vi "Digital Output User Interface.vi"() -> ()   [LabVIEW 2023, in "GUI.lvlib" / "Diagnostic.lvlib"]
uses:
  Diagnostic.lvlib
  Control/Digital Output 6514.ctl
  Control/Digital Output.ctl
  HardwareAbstractionLayer_LVOOP/Digital Output/NI Digital Output_class/NI Digital Output.lvclass
  D:/eDCU LTT/VT LTT Project/Source Code/HardwareAbstractionLayer_LVOOP/Digital Output/DO_class/DO.lvclass
  HardwareAbstractionLayer_LVOOP/Database/SQL Public VI/Control/DB Options.ctl
  HardwareAbstractionLayer_LVOOP/Main/Class Ref.ctl
  HardwareAbstractionLayer_LVOOP/DMM/DMM.lvclass
  HardwareAbstractionLayer_LVOOP/Function Generator/Function Generator.lvclass
  HardwareAbstractionLayer_LVOOP/Oscilloscope/Oscilloscope.lvclass
  HardwareAbstractionLayer_LVOOP/PowerSupply/PowerSupply.lvclass
  HardwareAbstractionLayer_LVOOP/Teststand/Teststand.lvclass
  HardwareAbstractionLayer_LVOOP/Analog Output/AO/AO.lvclass
  HardwareAbstractionLayer_LVOOP/Analog Input/AI/AI.lvclass
  HardwareAbstractionLayer_LVOOP/Database/Database.lvclass
  HardwareAbstractionLayer_LVOOP/Digital Output/DO_class/DO.lvclass
  HardwareAbstractionLayer_LVOOP/Digital Input/DI_class/DI.lvclass
  HardwareAbstractionLayer_LVOOP/PWM Output/PWM Output_class/PWM Output.lvclass
  HardwareAbstractionLayer_LVOOP/PWM Input/PWM Input_class/PWM Input.lvclass
  HardwareAbstractionLayer_LVOOP/NI Switch/NISwitch_class/NISwitch.lvclass
  HardwareAbstractionLayer_LVOOP/Modbus/Modbus_class/Modbus.lvclass
  HardwareAbstractionLayer_LVOOP/CAN/CAN Lib/CAN_class/CAN.lvclass
  HardwareAbstractionLayer_LVOOP/Main/Main.lvclass
  <userlib>/_OpenG.lib/appcontrol/appcontrol.llb/openg_application_control.lvlib
panel:
  in  "Start Acquire":bool
  in  "Stop Acquire":bool
  out "error out":errorcluster
  in  "error in":errorcluster
  in  "Operation":enum32{"6514-PXI2Slot9"}(tab)
  in  "PXIe_6514":T1
  in  "Stop":bool caption="Blank"
  in  "Apply":bool caption="Blank"
  # "Digital Output"
  # "Device:"
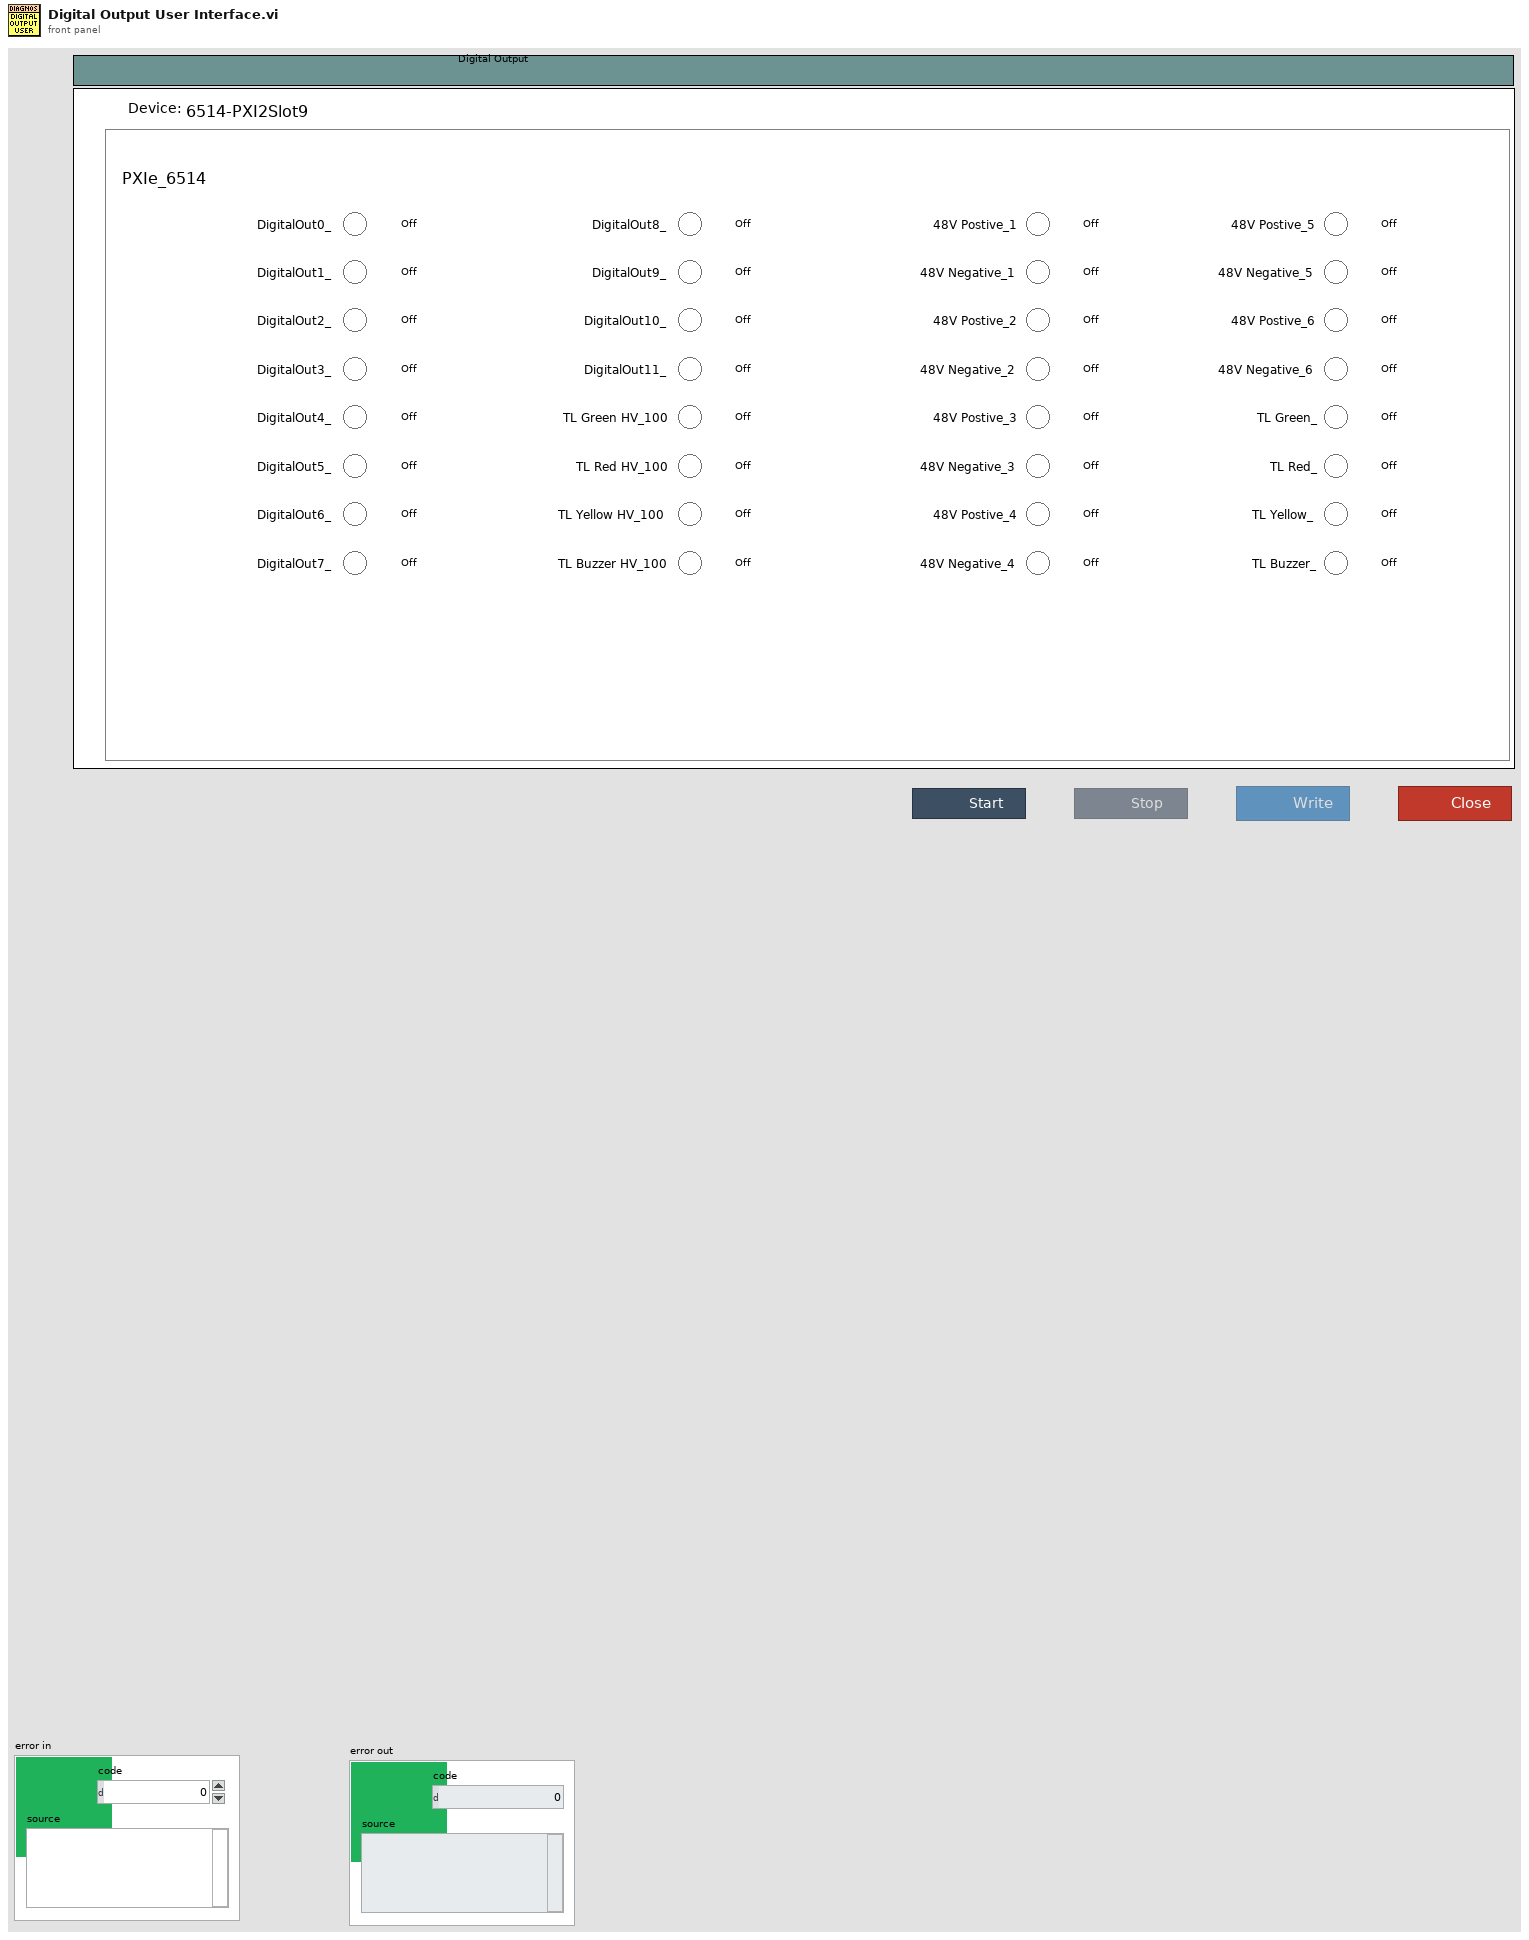
[diagram p1: front panel]
types:
  T1 = typedef "GUI.lvlib/Diagnostic.lvlib/Digital Output 6514.ctl" = cluster{"Channel-0":T2, "Channel-1":T2, "Channel-2":T2, "Channel-3":T2, "Channel-4":T2, "Channel-5":T2, "Channel-6":T2, "Channel-7":T2, "Channel-8":T2, "Channel-9":T2, "Channel-10":T2, "Channel-11":T2, "Channel-12":T2, "Channel-13":T2, "Channel-14":T2, "Channel-15":T2, "Channel-16":T2, "Channel-17":T2, "Channel-18":T2, "Channel-19":T2, "Channel-20":T2, "Channel-21":T2, "Channel-22":T2, "Channel-23":T2, "Channel-24":T2, "Channel-25":T2, "Channel-26":T2, "Channel-27":T2, "Channel-28":T2, "Channel-29":T2, "Channel-30":T2, "Channel-31":T2}
  T2 = typedef "GUI.lvlib/Diagnostic.lvlib/Digital Output.ctl" = bool
  T3 = typedef "HardwareAbstractionLayer_LVOOP.lvlib/Database.lvclass/DB Options.ctl" = enum16{"Init", "Select Data", "Insert Data", "Update Data", "Delete Data", "Execute Query", "Create Schema", "Create Table", "List Tables", "List Columns", "Close"}
  T4 = typedef "HardwareAbstractionLayer_LVOOP.lvlib/Main.lvclass/Class Ref.ctl" = cluster{"DMM":refnum<class "DMM.lvclass">, "Function Generator":refnum<class "Function Generator.lvclass">, "Oscilloscope":refnum<class "Oscilloscope.lvclass">, "PowerSupply":refnum<class "PowerSupply.lvclass">, "Teststand":refnum<class "Teststand.lvclass">, "AO":refnum<class "AO.lvclass">, "AI":refnum<class "AI.lvclass">, "Database":refnum<class "Database.lvclass">, "AO Waveform Generation":refnum<class "AO.lvclass">, "DO":refnum<class "DO.lvclass">, "DI":refnum<class "DI.lvclass">, "PWM Output":refnum<class "PWM Output.lvclass">, "PWM Input":refnum<class "PWM Input.lvclass">, "RelayOutput":refnum<class "NISwitch.lvclass">, "Modbus":refnum<class "Modbus.lvclass">, "CAN":refnum<class "CAN.lvclass">}
  T5 = enum8{"Enabled", "Disabled", "Disabled and Grayed Out"}
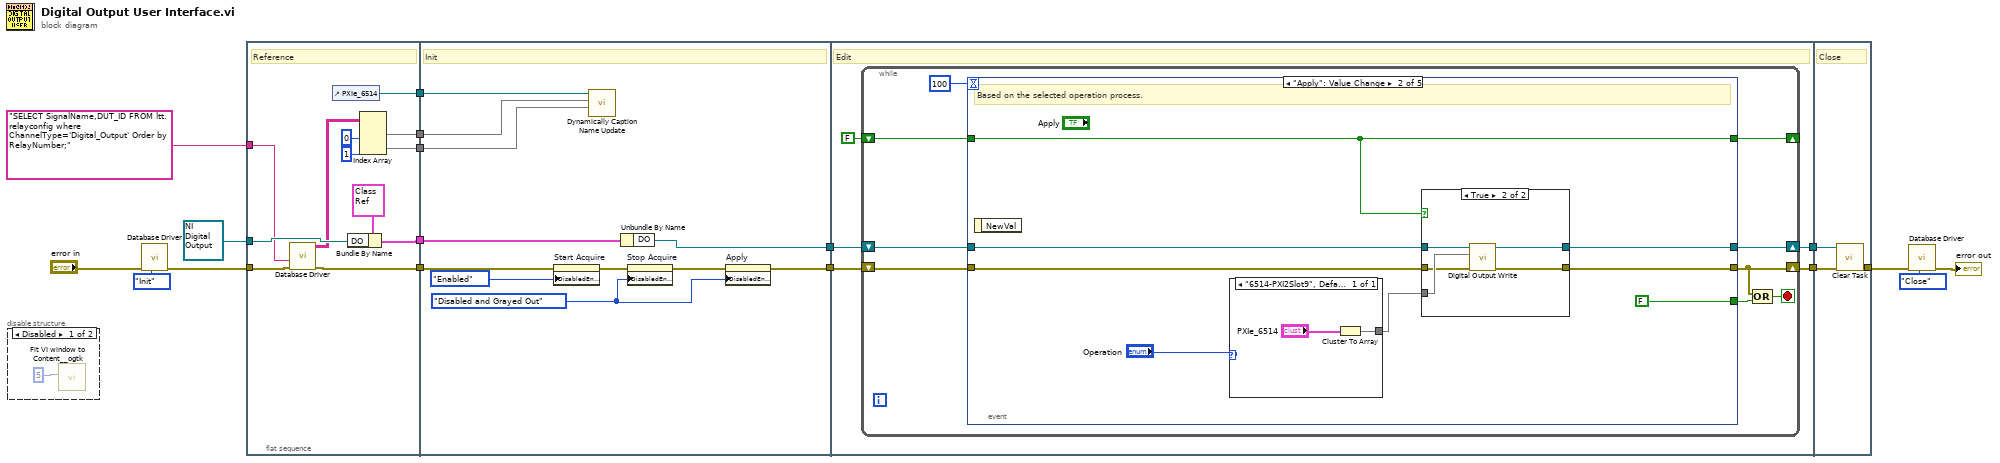
[diagram p0: block diagram]
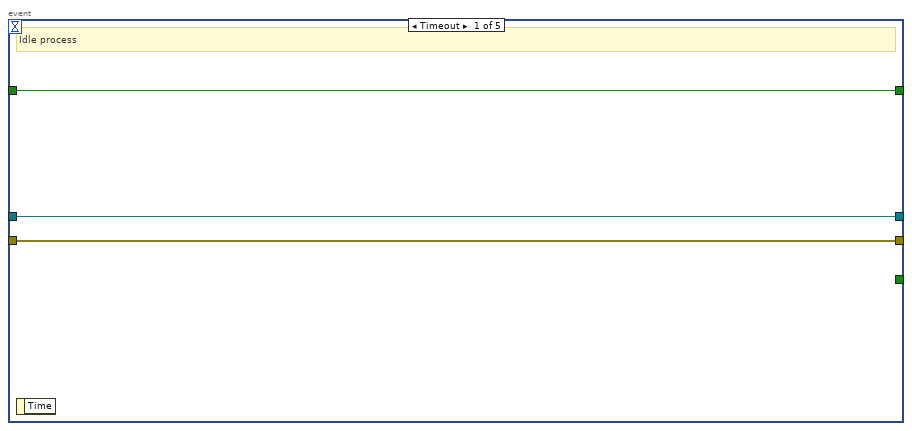
[diagram p3: hidden frame]
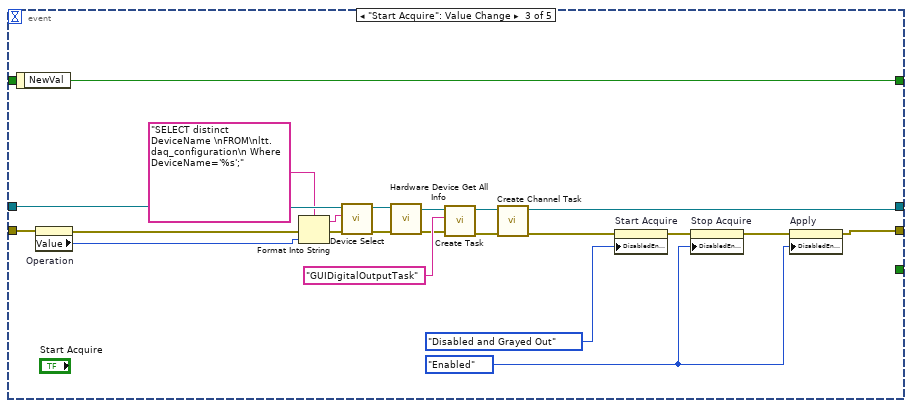
[diagram p5: hidden frame]
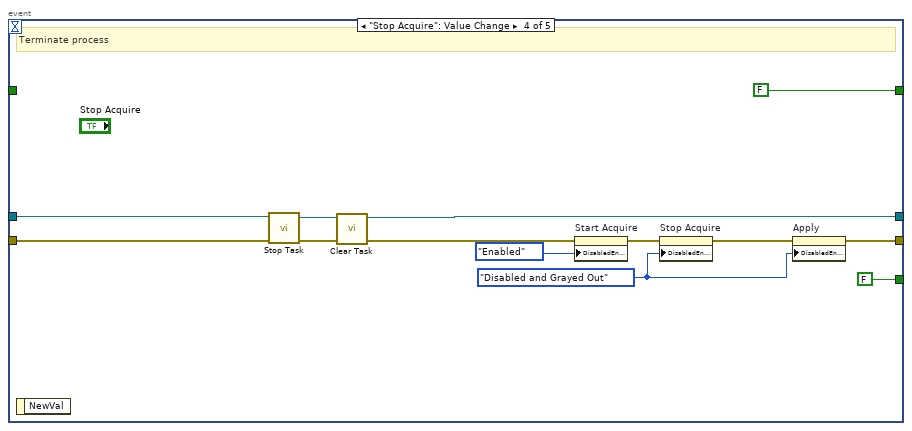
[diagram p6: hidden frame]
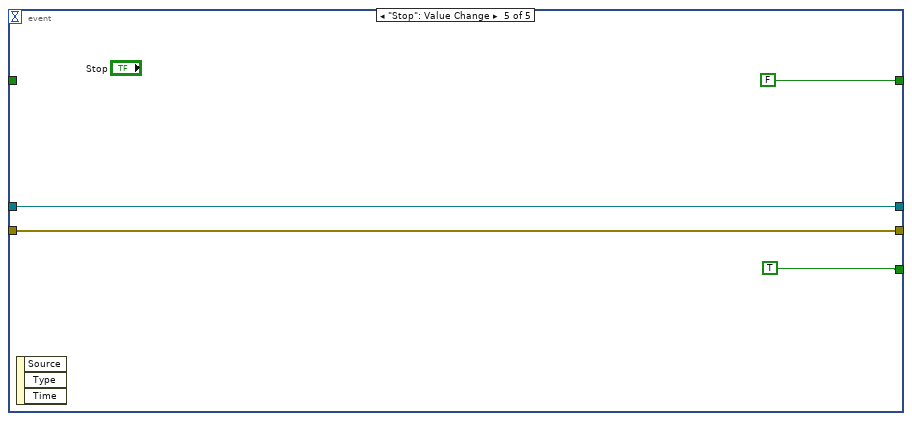
[diagram p7: hidden frame]
diagram:
  n1 = disable-structure shown="Disabled" {
    frame Disabled {
      n2 = call <userlib>:"Fit VI window to Content__ogtk.vi"("border spacing (2 px)"=5) -> ()  [unwired: 5 in, 2 out]
    }
    frame Enabled {
    }
  }
  n3 = call "Database Driver.vi"("Options"=DB_Options."Init", "error in"="error in") -> ("error out"=w8:errorcluster)  [unwired: 6 in, 3 out]
  n4 = flat-sequence {
    tunnel: [w29] -> w17
    tunnel: refnum<class "NI Digital Output.lvclass"> refnum ("HardwareAbstractionLayer_LVOOP.lvlib:NI Digital Output.lvclass") -> [w28]
    tunnel: w8 -> [w25]
    tunnel: [w24] -> w7
    tunnel: [w27] -> w4
    tunnel: "SELECT SignalName,DUT_ID FROM ltt.relayconfig where ChannelType='Digital_Output' Order by RelayNumber;" -> [w26]
    tunnel: [w21] -> w2
    tunnel: [w19] -> w1
    tunnel: w17 -> [w41]
    tunnel: [w40] -> w15
    tunnel: [w35] -> w9
    tunnel: w7 -> [w39]
    tunnel: w4 -> [w33]
    tunnel: w2 -> [w32]
    tunnel: w1 -> [w31]
    tunnel: w15 -> [w46]
    tunnel: [w44] -> w14
    tunnel: [w43] -> w13
    tunnel: w9 -> [w45]
    tunnel: w14 -> [w117]
    tunnel: w13 -> [w116]
    tunnel: [w115] -> w6
    frame #0 {
      # "Reference"
      n5 = call "Database Driver.vi"("error in"=w25, "SQL query"=w26) -> ("error out"=w24:errorcluster, "data"=w23:string[][])  [unwired: 6 in, 2 out]
      n6 = control-ref of="PXIe_6514"() -> (w27:refnum<vi>)
      n7 = Bundle By Name(cluster=T4 {"DMM"=refnum, "Function Generator"=refnum, "Oscilloscope"=refnum, "PowerSupply"=refnum, "Teststand"=refnum, "AO"=refnum, "AI"=refnum, "Database"=refnum, "AO Waveform Generation"=refnum, "DO"=refnum, "DI"=refnum, "PWM Output"=refnum, "PWM Input"=refnum, "RelayOutput"=refnum, "Modbus"=refnum, "CAN"=refnum} ("Class Cluster"), "DO"=w28) -> (w29:T4)
      n8 = Index Array(array=w23, index (col) #1=0 ("disabled index (col)"), index (col) #2=1 ("index (col)")) -> (element #1=w21:string[], element #2=w19:string[])  [unwired: 2 in]
    }
    frame #1 {
      w34 = T5."Disabled and Grayed Out" ("Disabled")
      # "Init"
      n9 = property on="Start Acquire" class="Bool"(error in=w39, "DisabledEnum"=T5."Enabled" ("Disabled")) -> (error out=w38:errorcluster)  [unwired: 1 in, 1 out]
      n10 = call "Dynamically Caption Name Update.vi"("DUT_Number"=w31, "Caption Name"=w32, "Clust Refnum"=w33) -> ()  [unwired: 8 in, 1 out]
      n11 = Unbundle By Name(w41) -> ("DO"=w40:refnum<class "DO.lvclass">)
      n12 = property on="Stop Acquire" class="Bool"(error in=w38, "DisabledEnum"=w34) -> (error out=w36:errorcluster)  [unwired: 1 in, 1 out]
      n13 = property on="Apply" class="Bool (strict)"(error in=w36, "DisabledEnum"=w34) -> (error out=w35:errorcluster)  [unwired: 1 in, 1 out]
    }
    frame #2 {
      # "Edit"
      n14 = while {
        shift-right: [w47] -> w43
        shift-left: w45 -> [w52]
        shift-right: [w51] -> w44
        shift-left: w46 -> [w53]
        shift-right: [w50] -> _
        shift-left: FALSE ("NewVal") -> [w49]
        stop <- w48 stop-if-true
        n15 = event shown="[1] \"Apply\": Value Change" {
          selector: _ -> [_ _ _ _ _]
          dyn-events: _ -> [_ _ _ _ _]
          timeout: 100 -> [_ _ _ _ _]
          tunnel: [_ FALSE _ FALSE TRUE] -> w55
          tunnel: w53 -> [w58 w61 w97 w107 w114]
          tunnel: w52 -> [w57 w60 w94 w108 w113]
          tunnel: [w58 w66 w96 w106 w114] -> w51
          tunnel: [w57 w65 w87 w101 w113] -> w47
          tunnel: [w56 w59 w95 FALSE ("NewVal") FALSE ("NewVal")] -> w50
          tunnel: w49 -> [w56 w59 _ _ _]
          event Timeout {
            # "Idle process"
            n16 = event-data() -> ()  [unwired: 1 in, 1 out]
          }
          event "Apply": Value Change {
            # "Based on the selected operation process."
            n17 = event-data() -> ()  [unwired: 1 in, 1 out]
            n18 = case shown="\"6514-PXI2Slot9\", Default" "Operation" {
              tunnel: [w74] -> w63
              frame "6514-PXI2Slot9", Default {
                n19 = Cluster To Array(cluster="PXIe_6514") -> (array=w74:T2[])
              }
            }
            n20 = case shown="True" w59 {
              tunnel: [w68 w73] -> w66
              tunnel: [w67 w72] -> w65
              tunnel: w63 -> [_ w71]
              tunnel: w61 -> [w68 w70]
              tunnel: w60 -> [w67 w69]
              frame False {
              }
              frame True {
                n21 = call-dynamic "Digital Output Write.vi"("error in (no error)"=w69, "Digital Output Write"=w71, "DO in"=w70) -> ("error out"=w72:errorcluster, "DO out"=w73:refnum<class "DO.lvclass">)  [unwired: 7 in]
              }
            }
          }
          event "Start Acquire": Value Change {
            w86 = T5."Enabled" ("Disabled")
            n22 = event-data() -> ("NewVal"=w95:bool)  [unwired: 1 in]
            n23 = property on="Operation" class="TabCtl (strict)"(error in=w94) -> (error out=w93:errorcluster, "Value"=w92:enum32{"6514-PXI2Slot9"})  [unwired: 1 in, 1 out]
            n24 = Format Into String(format string="SELECT distinct DeviceName \nFROM\nltt.daq_configuration\n Where DeviceName='%s';" ("SQL query"), error in=w93, w92) -> (resulting string=w82:string, error out=w84:errorcluster)  [unwired: 1 in]
            n25 = call-dynamic "Device Select.vi"("error in (no error)"=w84, "SQL query"=w82, "DO in"=w97) -> ("error out"=w80:errorcluster, "DO out"=w81:refnum<class "DO.lvclass">)  [unwired: 7 in]
            n26 = call-dynamic "Hardware Device Get All Info.vi"("error in (no error)"=w80, "DO in"=w81) -> ("error out"=w79:errorcluster, "DO out"=w78:refnum<class "DO.lvclass">)  [unwired: 8 in]
            n27 = call-dynamic "Create Task.vi"("error in (no error)"=w79, "Task Name"="GUIDigitalOutputTask", "DO in"=w78) -> ("error out"=w76:errorcluster, "DO out"=w77:refnum<class "DO.lvclass">)  [unwired: 7 in]
            n28 = call-dynamic "Create Channel Task.vi"("error in (no error)"=w76, "DO in"=w77) -> ("error out"=w89:errorcluster, "DO out"=w96:refnum<class "DO.lvclass">)  [unwired: 8 in]
            n29 = property on="Start Acquire" class="Bool"(error in=w89, "DisabledEnum"=T5."Disabled and Grayed Out" ("Disabled")) -> (error out=w90:errorcluster)  [unwired: 1 in, 1 out]
            n30 = property on="Stop Acquire" class="Bool"(error in=w90, "DisabledEnum"=w86) -> (error out=w88:errorcluster)  [unwired: 1 in, 1 out]
            n31 = property on="Apply" class="Bool (strict)"(error in=w88, "DisabledEnum"=w86) -> (error out=w87:errorcluster)  [unwired: 1 in, 1 out]
          }
          event "Stop Acquire": Value Change {
            w100 = T5."Disabled and Grayed Out" ("Disabled")
            # "Terminate process"
            n32 = event-data() -> ()  [unwired: 1 in, 1 out]
            n33 = call-dynamic "Stop Task.vi"("error in (no error)"=w108, "DO in"=w107) -> ("error out"=w98:errorcluster, "DO out"=w99:refnum<class "DO.lvclass">)  [unwired: 8 in]
            n34 = call-dynamic "Clear Task.vi"("error in (no error)"=w98, "DO in"=w99) -> ("error out"=w103:errorcluster, "DO out"=w106:refnum<class "DO.lvclass">)  [unwired: 8 in]
            n35 = property on="Start Acquire" class="Bool"(error in=w103, "DisabledEnum"=T5."Enabled" ("Disabled")) -> (error out=w104:errorcluster)  [unwired: 1 in, 1 out]
            n36 = property on="Stop Acquire" class="Bool"(error in=w104, "DisabledEnum"=w100) -> (error out=w102:errorcluster)  [unwired: 1 in, 1 out]
            n37 = property on="Apply" class="Bool (strict)"(error in=w102, "DisabledEnum"=w100) -> (error out=w101:errorcluster)  [unwired: 1 in, 1 out]
          }
          event "Stop": Value Change {
            n38 = event-data() -> ()  [unwired: 1 in, 3 out]
          }
        }
        n39 = Compound Arithmetic op=OR(w47, w55) -> (w48:bool)
      }
    }
    frame #3 {
      # "Close"
      n40 = call-dynamic "Clear Task.vi"("error in (no error)"=w116, "DO in"=w117) -> ("error out"=w115:errorcluster)  [unwired: 8 in, 1 out]
    }
  }
  n41 = call "Database Driver.vi"("Options"=DB_Options."Close", "error in"=w6) -> ("error out"=→"error out":errorcluster)  [unwired: 6 in, 3 out]
